vi "start_sweep.vi"(8 "error in (no error)":errorcluster, 11 "ScanModeMG090624Camera in":refnum<class "ImagingModeMG090624Camera.lvclass">) -> (0 "error out":errorcluster, 3 "ScanModeMG090624Camera out":refnum<class "ImagingModeMG090624Camera.lvclass">)   [LabVIEW 2010, in "ImagingModeMG090624Camera.lvclass"]
uses:
  ImagingModeMG090624Camera.lvclass
  ImagingModeMG090624Camera.lvclass/ImagingModeMG090624Camera.ctl
  ImagingModeDL091001Scaffold/ImagingModeDL091001Scaffold/ImagingModeDL091001Scaffold.lvclass
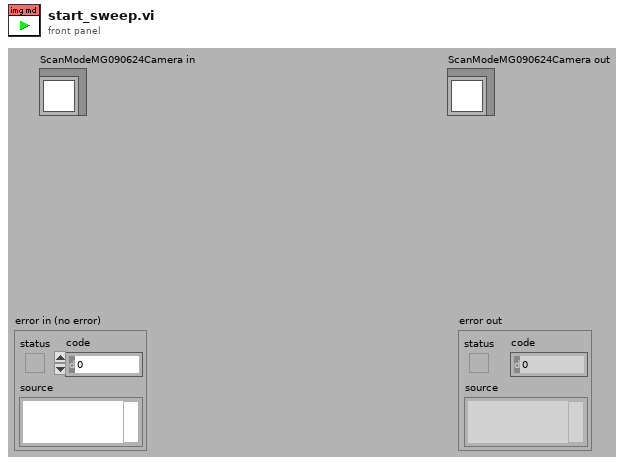
[diagram p1: front panel]
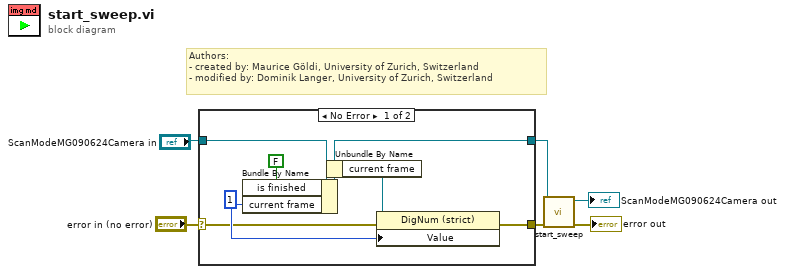
[diagram p0: block diagram]
diagram:
  # "Authors: \n- created by: Maurice Göldi, University of Zurich, Switzerland\n- modified by: Dominik Langer, University of Zurich, Switzerland"
  n1 = case shown="No Error" "error in (no error)" {
    selector: "error in (no error)" -> [w9 w15]
    tunnel: [w8 w15] -> w3
    tunnel: [w12 w14] -> w1
    tunnel: "ScanModeMG090624Camera in" -> [w13 w14]
    frame No Error {
      w10 = 1
      n2 = Bundle By Name(cluster=w13, "is finished"=FALSE, "current frame"=w10) -> (w12:refnum<class "ImagingModeMG090624Camera.lvclass">)
      n3 = Unbundle By Name(w12) -> ("current frame"=w11:refnum<vi>)
      n4 = property class="DigNum (strict)"(reference=w11, error in=w9, "Value"=w10) -> (error out=w8:errorcluster)  [unwired: 1 out]
    }
    frame Error {
    }
  }
  n5 = call-parent "start_sweep.vi"("error in (no error)"=w3, "ScanModeDL091001Scaffold in"=w1) -> ("error out"=→"error out":errorcluster, "ScanModeDL091001Scaffold out"=→"ScanModeMG090624Camera out":refnum<class "ImagingModeMG090624Camera.lvclass">)  [unwired: 8 in]
